vi "Calculate Current Read Size.vi"(10 "Size Remaining in":i64, 11 "Total Size":i64) -> (1 "Stop":bool, 2 "Size Remaining out":i64, 4 "Current Read Size":i64, 6 "Offset":i64)   [LabVIEW 2010, in "TDMS to ASCII Convert.lvlib"]
uses:
  TDMS to ASCII Convert.lvlib
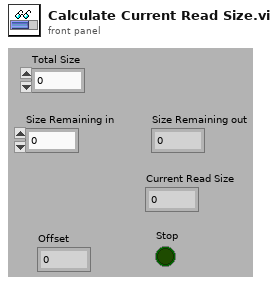
[diagram p1: front panel]
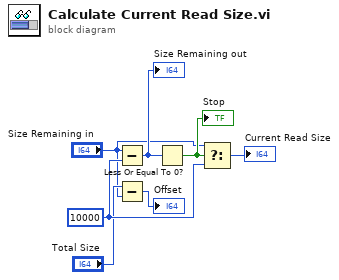
[diagram p0: block diagram]
diagram:
  w4 = i64 10000 ("y")
  n1 = Subtract(x="Size Remaining in", y=w4) -> (x-y=w6:i64)
  "Size Remaining out" <- w6
  n2 = Subtract(x="Total Size", y="Size Remaining in") -> (x-y=→"Offset":i64)
  n3 = Less Or Equal To 0?(x=w6) -> (x <= 0?=w7:bool)
  "Stop" <- w7
  n4 = Select(t="Size Remaining in", s=w7, f=w4) -> (s? t:f=→"Current Read Size":i64)
